vi "main.vi"() -> ()   [LabVIEW 2025]
uses:
  Controls/States.ctl
  Controls/HR_Data_Structure.ctl
  Controls/Raw_Data_IN_HR.ctl
  Controls/Runner_Data_Structure.ctl
panel:
  out "BPM":cluster{"Time":timestamp[], "Bpm":i32[]}(graph)
  out "Zone PLOT":T1(graph)
  out "Zone Data":string[][](array[string]) caption="HEART RATE ZONES"
  in  "File Path":path
  out "error out":errorcluster
  in  "error in":errorcluster
  in  "Stop":bool
  in  "Save Results":bool
  in  "New Training":bool
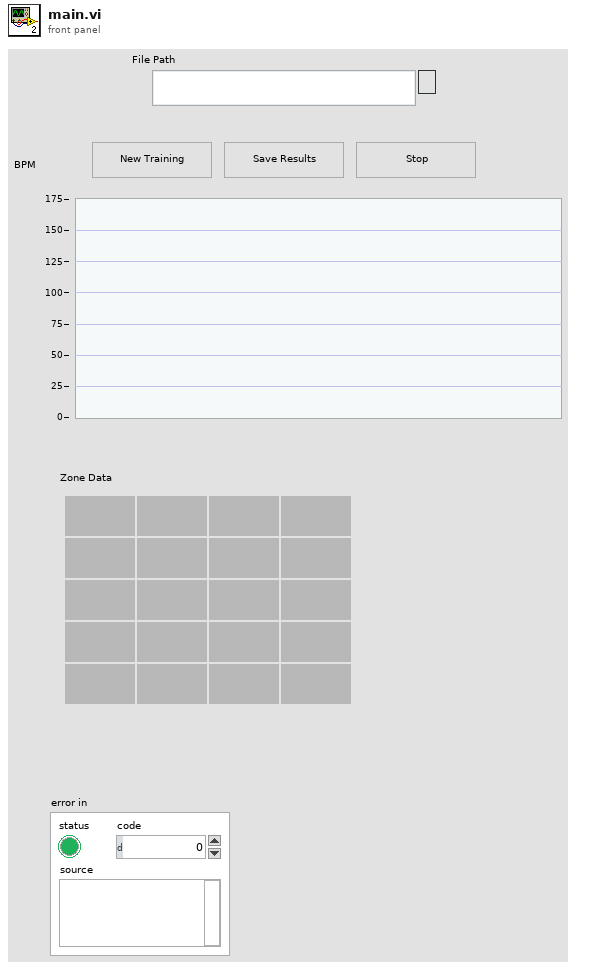
[diagram p1: front panel]
types:
  T1 = cluster{"Total Time in Zone":dbl[], "Heart Rate Zone No":dbl[]}
  T2 = typedef "HR_Data_Structure.ctl" = cluster{"HR Max":i32, "% HR MAX ":dbl[], "Raw Data":T3, "Runner's Data":T4, "HR Zone":string[][], "Total Time in Zone":dbl[], "Heart Rate Zone No":dbl[]}
  T3 = typedef "Raw_Data_IN_HR.ctl" = cluster{"Time":timestamp[], "Bpm":i32[]}
  T4 = typedef "Runner_Data_Structure.ctl" = cluster{"Name":string, "Age":i32}
  T5 = typedef "States.ctl" = enum16{"Application Error", "Init", "Idle", "Analyse New Training", "Save", "Error Handling", "Stop"}
  T6 = enum16{"open", "replace", "create", "open or create", "replace or create", "replace or create with confirmation"}
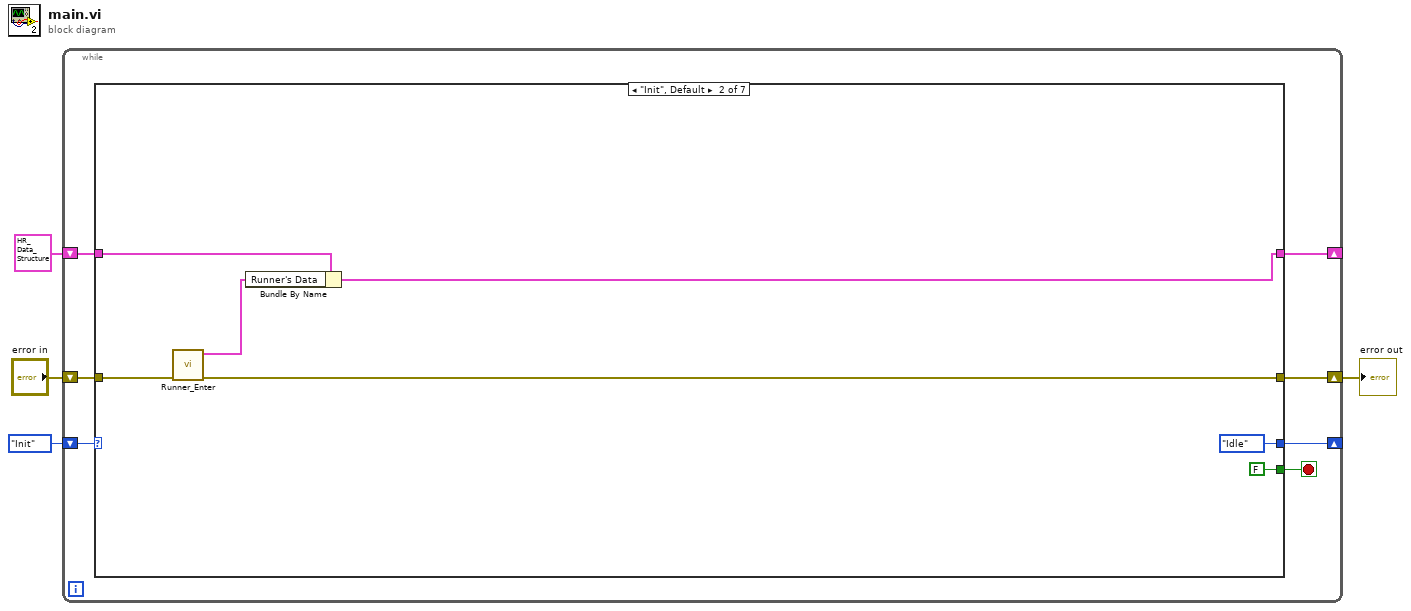
[diagram p0: block diagram]
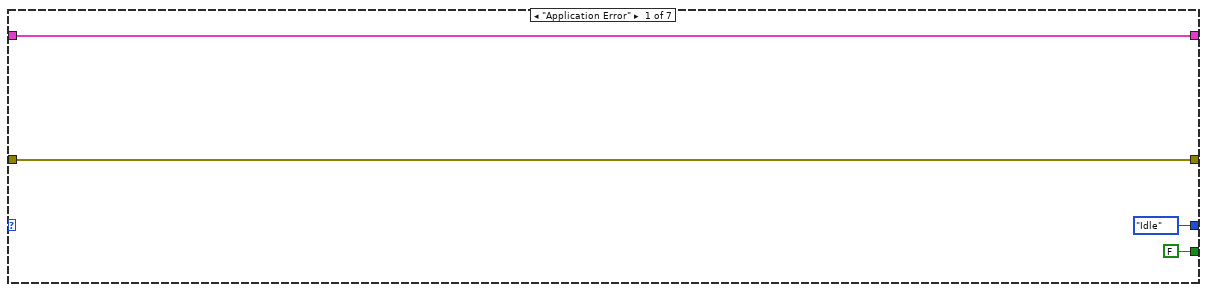
[diagram p2: hidden frame]
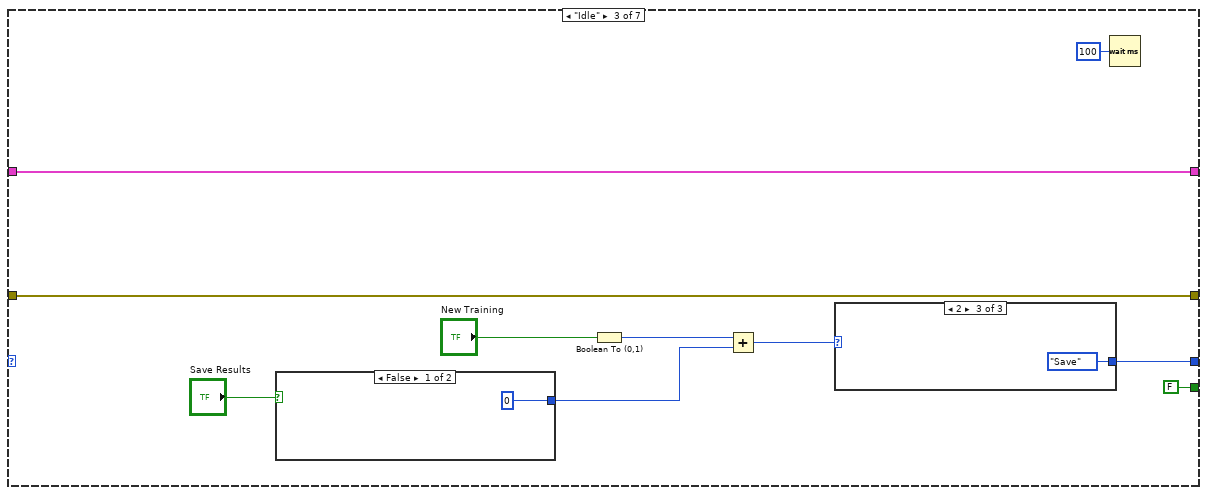
[diagram p3: hidden frame]
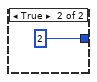
[diagram p4: hidden frame]
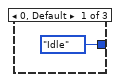
[diagram p5: hidden frame]
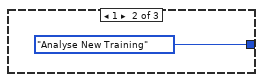
[diagram p6: hidden frame]
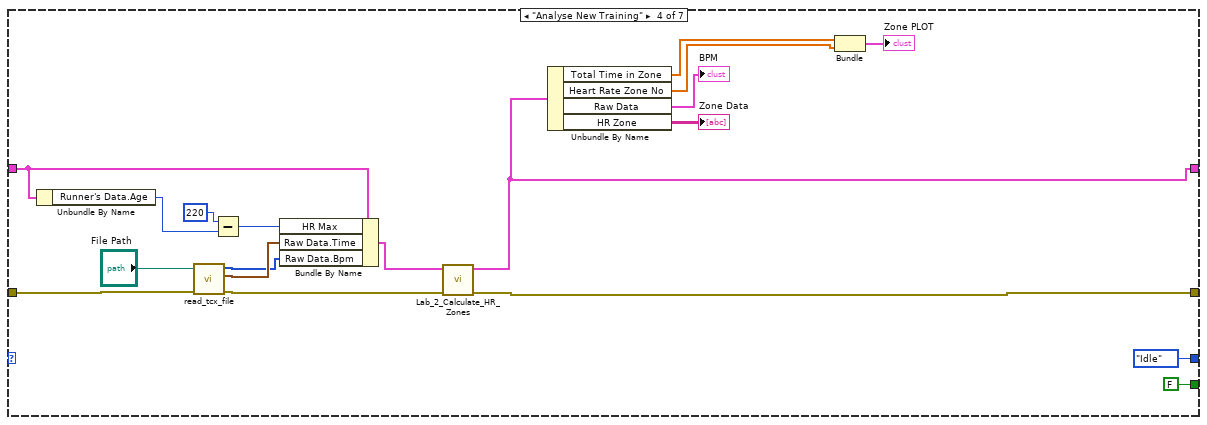
[diagram p7: hidden frame]
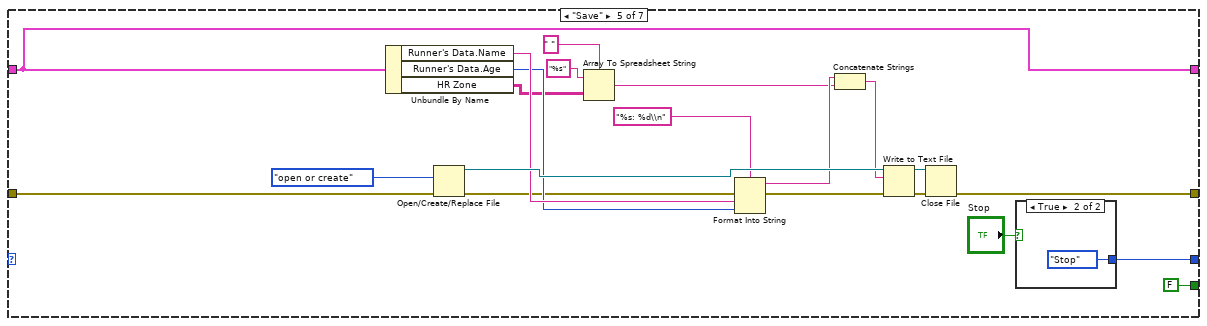
[diagram p8: hidden frame]
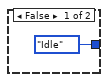
[diagram p9: hidden frame]
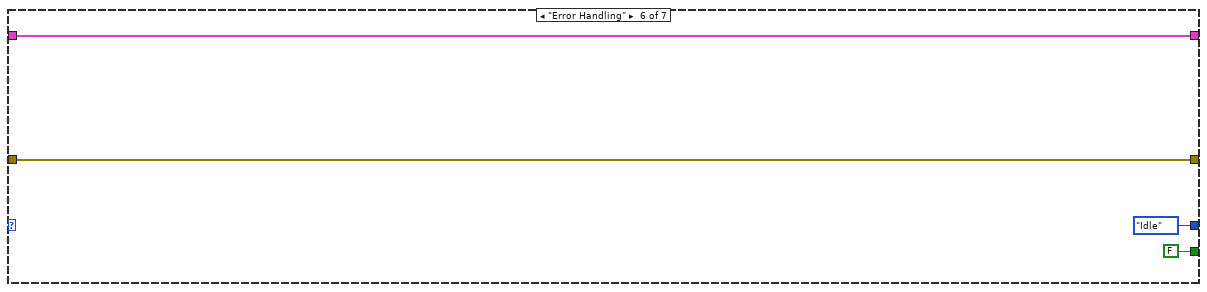
[diagram p10: hidden frame]
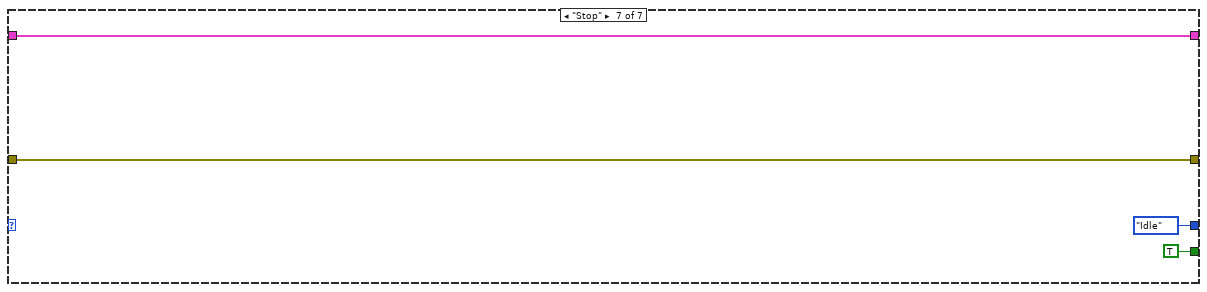
[diagram p11: hidden frame]
diagram:
  n1 = while {
    shift-right: [w11] -> _
    shift-left: States."Init" -> [w5]
    shift-right: [w8] -> _
    shift-left: T2 data[18004B] ("HR Data Structure 2") -> [w7]
    shift-right: [w9] -> w2
    shift-left: "error in" -> [w10]
    stop <- w6 stop-if-true
    n2 = case shown="\"Init\", Default" w5 {
      tunnel: [States."Idle" States."Idle" w29 States."Idle" w69 States."Idle" States."Idle"] -> w11
      tunnel: w10 -> [w13 w20 w28 w44 w75 w82 w86]
      tunnel: [w13 w19 w28 w56 w72 w82 w86] -> w9
      tunnel: [w14 w18 w26 w38 w71 w83 w85] -> w8
      tunnel: w7 -> [w14 w16 w26 w39 w71 w83 w85]
      tunnel: [FALSE FALSE FALSE FALSE FALSE FALSE TRUE] -> w6
      frame "Application Error" {
      }
      frame "Init", Default {
        n3 = call "Runner_Enter.vi"("error in"=w20) -> ("error out"=w19:errorcluster, "Runner's Data OUT"=w22:T4)  [unwired: 9 in]
        n4 = Bundle By Name(cluster=w16, "Runner's Data"=w22) -> (w18:T2)
      }
      frame "Idle" {
        n5 = case shown="False" "Save Results" {
          tunnel: [0 2] -> w24
          frame False {
          }
          frame True {
          }
        }
        n6 = Boolean To (0,1)(Boolean="New Training") -> (0, 1=w30:i16)
        n7 = Add(x=w30, y=w24) -> (x+y=w31:i32)
        n8 = case shown="2" w31 {
          tunnel: [States."Idle" States."Analyse New Training" States."Save"] -> w29
          frame 0, Default {
          }
          frame 1 {
          }
          frame 2 {
          }
        }
        n9 = Wait (ms)(milliseconds to wait=u32 100) -> ()  [unwired: 1 out]
      }
      frame "Analyse New Training" {
        n10 = Unbundle By Name(w39) -> ("Runner's Data.Age"=w54:i32)
        n11 = call "read_tcx_file.vi"("error in"=w44, "File Path"="File Path") -> ("error out"=w43:errorcluster, "Time"=w42:timestamp[], "Bmp"=w41:i32[])  [unwired: 7 in]
        n12 = Subtract(x=220, y=w54) -> (x-y=w52:i32)
        n13 = Bundle By Name(cluster=w39, "HR Max"=w52, "Raw Data.Time"=w42, "Raw Data.Bpm"=w41) -> (w51:T2)
        n14 = call "Lab_2_Calculate_HR_Zones.vi"("Error IN"=w43, "HR Data Structure IN"=w51) -> ("Error OUT"=w56:errorcluster, "HR Data Structure OUT"=w38:T2)  [unwired: 8 in]
        n15 = Unbundle By Name(w38) -> ("Total Time in Zone"=w45:dbl[], "Heart Rate Zone No"=w46:dbl[], "Raw Data"=→"BPM":T3, "HR Zone"=→"Zone Data":string[][])
        n16 = Bundle("Total Time in Zone"=w45, "Heart Rate Zone No"=w46) -> (→"Zone PLOT":T1)  [unwired: 1 in]
      }
      frame "Save" {
        n17 = Unbundle By Name(w71) -> ("Runner's Data.Name"=w66:string, "Runner's Data.Age"=w65:i32, "HR Zone"=w62:string[][])
        n18 = Open/Create/Replace File(error in=w75, operation (0:open)=T6."open or create") -> (refnum out=w76:refnum<file>, error out=w64:errorcluster)  [unwired: 4 in, 1 out]
        n19 = Array To Spreadsheet String(delimiter (Tab)=" ", array=w62, 3:"%s" ("format string")) -> (spreadsheet string=w60:string)
        n20 = Format Into String(format string="%s: %d\\n", error in=w64, w66, w65) -> (resulting string=w61:string, error out=w63:errorcluster)  [unwired: 1 in]
        n21 = Concatenate Strings(w61, w60) -> (w59:string)
        n22 = Write to Text File(file (use dialog)=w76, text=w59, error in=w63) -> (refnum out=w74:refnum<file>, error out=w73:errorcluster)  [unwired: 1 in, 1 out]
        n23 = Close File(refnum=w74, error in=w73) -> (error out=w72:errorcluster)  [unwired: 1 out]
        n24 = case shown="True" "Stop" {
          tunnel: [States."Idle" States."Stop"] -> w69
          frame False {
          }
          frame True {
          }
        }
      }
      frame "Error Handling" {
      }
      frame "Stop" {
      }
    }
  }
  "error out" <- w2
